vi "NearestNeighbor.vi"(6 "Algorithm":enum16{"RRT", "A*"}(ring), 8 "k":i32=2, 9 "Depth":i32=1, 10 "index":i32, 11 "KD Tree":dbl[][](array[numeric])) -> ()   [LabVIEW 2016]
uses:
  <vilib>/Analysis/_algsub.llb/Real Vector Norm.vi
  NearestGlobal.vi
  NearestDistanceGlobal.vi
  <vilib>/Analysis/NI_AALPro.lvlib
panel:
  out "Current Dimention":i32
  in  "target":dbl[](array[numeric])
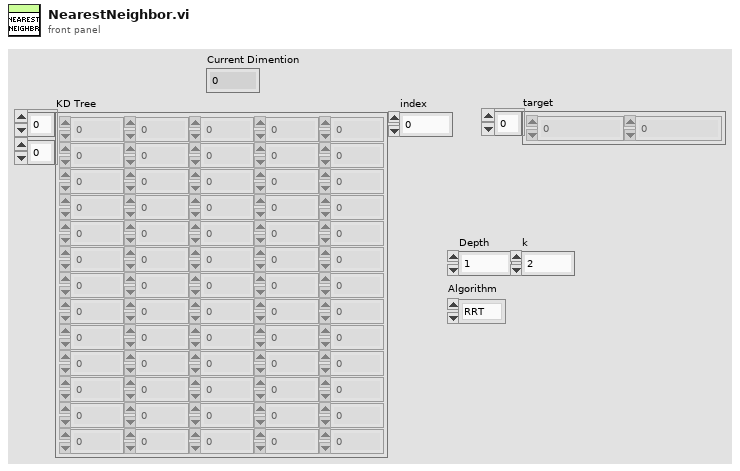
[diagram p1: front panel]
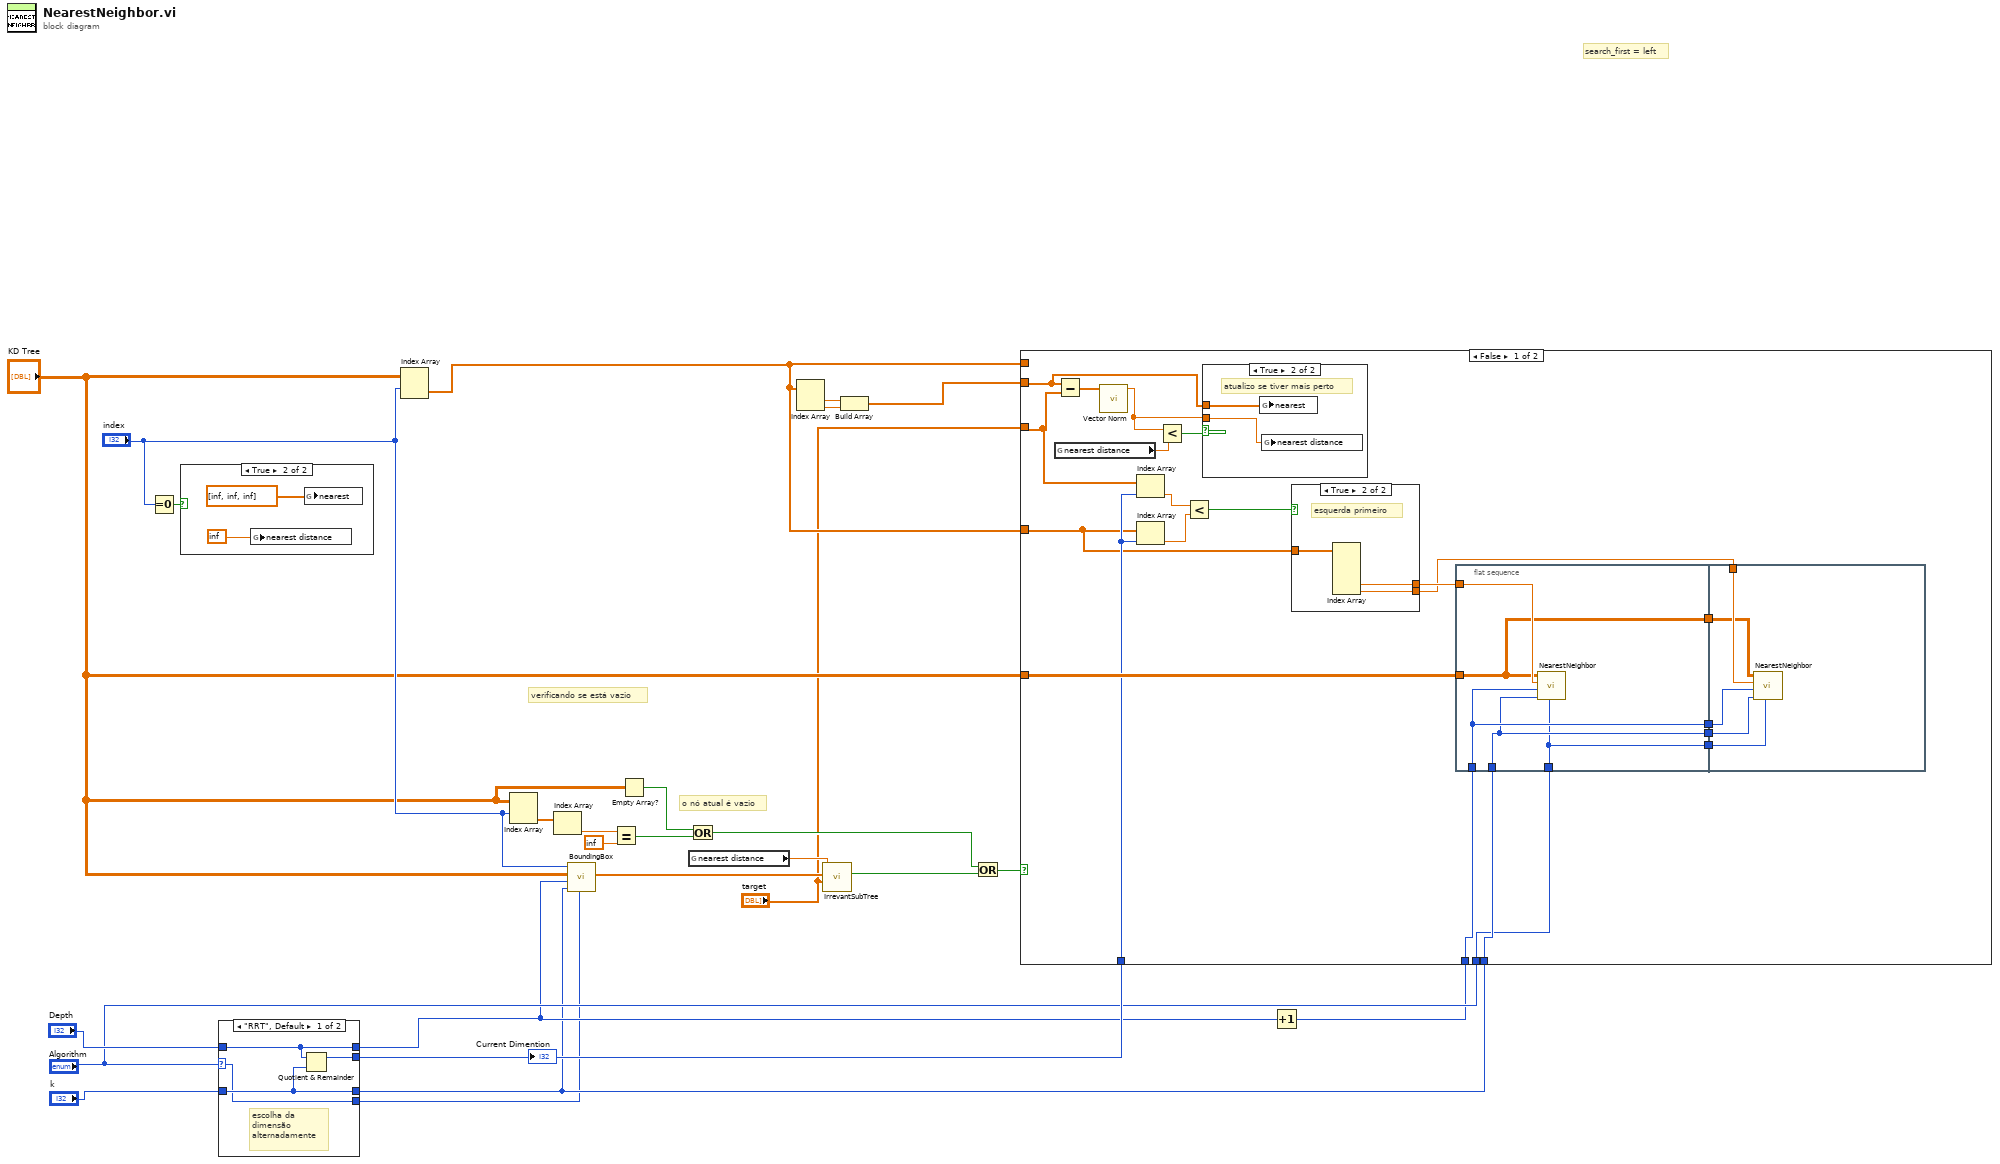
[diagram p0: block diagram]
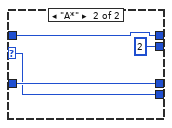
[diagram p3: hidden frame]
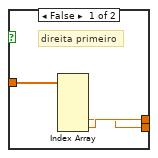
[diagram p4: hidden frame]
diagram:
  # "o nó atual é vazio"
  # "search_first = left"
  # "verificando se está vazio"
  n1 = Equal To 0?(x="index") -> (x = 0?=w6:bool)
  n2 = case shown="True" w6 {
    frame False {
    }
    frame True {
      n3 = global write "NearestDistanceGlobal.vi" "nearest distance"(inf) -> ()
      n4 = global write "NearestGlobal.vi" "nearest"(dbl[] [inf, inf, inf] ("target")) -> ()
    }
  }
  n5 = case shown="\"RRT\", Default" "Algorithm" {
    selector: "Algorithm" -> [w29 w33]
    tunnel: [w32 2] -> w24
    tunnel: [w31 w34] -> w18
    tunnel: [w30 w36] -> w17
    tunnel: "Depth" -> [w31 w34]
    tunnel: "k" -> [w30 w36]
    tunnel: [w29 w33] -> w16
    frame "RRT", Default {
      # "escolha da \ndimensão \nalternadamente"
      n6 = Quotient & Remainder(x=w31, y=w30) -> (x-y*floor(x/y)=w32:i32)  [unwired: 1 out]
    }
    frame "A*" {
    }
  }
  "Current Dimention" <- w24
  n7 = Index Array(array="KD Tree", index (row)="index") -> (element=w10:dbl[])  [unwired: 1 in]
  n8 = Index Array(array="KD Tree", index (row)="index") -> (element=w19:dbl[])  [unwired: 1 in]
  n9 = Index Array(array=w19) -> (element=w4:dbl)  [unwired: 1 in]
  n10 = call "BoundingBox.vi"("Algorithm"=w16, "k"=w17, "Depth"=w18, "Tree"="KD Tree", "index"="index") -> ("Bounding Box"=w8:dbl[])  [unwired: 6 in]
  n11 = Equal?(x=w4, y=inf) -> (x = y?=w20:bool)
  n12 = Empty Array?(array="KD Tree") -> (empty?=w21:bool)
  n13 = global read "NearestDistanceGlobal.vi" "nearest distance"() -> (w9:dbl)
  n14 = Or(x=w21, y=w20) -> (x .or. y?=w11:bool)
  n15 = Index Array(array=w10) -> (element #1=w15:dbl, element #2=w14:dbl)  [unwired: 2 in]
  n16 = call "IrrevantSubTree.vi"("best dist"=w9, "Bounding Box"=w8, "target"="target") -> ("Irrelevant subTree"=w7:bool)  [unwired: 7 in]
  n17 = Build Array(w15, w14) -> (w13:dbl[])
  n18 = Or(x=w11, y=w7) -> (x .or. y?=w12:bool)
  n19 = Increment(x=w18) -> (x+1=w22:i32)
  n20 = case shown="False" w12 {
    tunnel: w10 -> [_ _]
    tunnel: w24 -> [w50 _]
    tunnel: w22 -> [w43 _]
    tunnel: w17 -> [w40 _]
    tunnel: "Algorithm" -> [w38 _]
    tunnel: "target" -> [w51 _]
    tunnel: w13 -> [w54 _]
    tunnel: "KD Tree" -> [w52 _]
    tunnel: w10 -> [w46 _]
    frame False {
      n21 = global read "NearestDistanceGlobal.vi" "nearest distance"() -> (w55:dbl)
      n22 = Subtract(x=w54, y=w51) -> (x-y=w57:dbl[])
      n23 = call-poly <vilib>:"Vector Norm.vi"("Input Vector"=w57) -> ("norm"=w53:dbl)  [unwired: 9 in, 1 out]
      n24 = Index Array(array=w51, index=w50) -> (element=w49:dbl)
      n25 = Index Array(array=w46, index=w50) -> (element=w48:dbl)
      n26 = Less?(x=w53, y=w55) -> (x < y?=w56:bool)
      n27 = Less?(x=w49, y=w48) -> (x < y?=w47:bool)
      n28 = case shown="True" w56 {
        tunnel: w54 -> [_ w75]
        tunnel: w53 -> [_ w74]
        frame False {
        }
        frame True {
          # "atualizo se tiver mais perto"
          n29 = global write "NearestGlobal.vi" "nearest"(w75) -> ()
          n30 = global write "NearestDistanceGlobal.vi" "nearest distance"(w74) -> ()
        }
      }
      n31 = case shown="True" w47 {
        tunnel: w46 -> [w70 w73]
        tunnel: [w69 w72] -> w45
        tunnel: [w68 w71] -> w44
        frame False {
          # "direita primeiro"
          n32 = Index Array(array=w70) -> (element #4=w68:dbl, element #5=w69:dbl)  [unwired: 5 in, 3 out]
        }
        frame True {
          # "esquerda primeiro"
          n33 = Index Array(array=w73) -> (element #4=w72:dbl, element #5=w71:dbl)  [unwired: 5 in, 3 out]
        }
      }
      n34 = flat-sequence {
        tunnel: w52 -> [w60]
        tunnel: w45 -> [w62]
        tunnel: w43 -> [w61]
        tunnel: [w61] -> w42
        tunnel: [w60] -> w41
        tunnel: w40 -> [w59]
        tunnel: [w59] -> w39
        tunnel: w38 -> [w58]
        tunnel: [w58] -> w37
        tunnel: w44 -> [w66]
        tunnel: w42 -> [w67]
        tunnel: w41 -> [w65]
        tunnel: w39 -> [w64]
        tunnel: w37 -> [w63]
        frame #0 {
          n35 = call "NearestNeighbor.vi"("Algorithm"=w58, "k"=w59, "Depth"=w61, "index"=w62, "KD Tree"=w60) -> ()  [unwired: 7 in]
        }
        frame #1 {
          n36 = call "NearestNeighbor.vi"("Algorithm"=w63, "k"=w64, "Depth"=w67, "index"=w66, "KD Tree"=w65) -> ()  [unwired: 7 in]
        }
      }
    }
    frame True {
      # "mantenho o mesmo nearest de sempre"
      # "A distancia aos limites já é maior q a minha melhor distância"
      # "nem olho está sub árvore"
    }
  }
